vi "Initialize_Map.vi"(0 "Object_Data_In":T1, 5 "Default_Data":map{string, refnum<class "Calculator.lvclass">}(c390), 9 "Class_Names":string[](array[string])) -> (4 "Object_Data_Out":T1)   [LabVIEW 2021]
doc: "Used to initialize the map"
uses:
  Classes/Calculator/Calculator.lvclass
  Controls/Object_Data.ctl
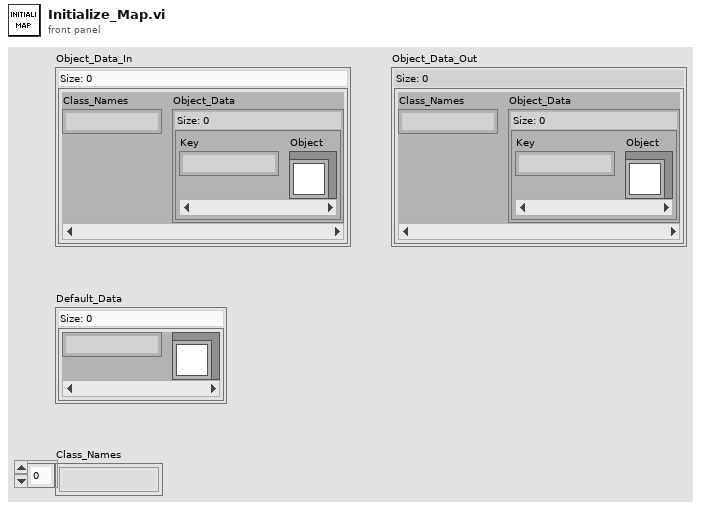
[diagram p1: front panel]
types:
  T1 = typedef "Object_Data.ctl" = map{string, map{string, refnum<class "Calculator.lvclass">}}
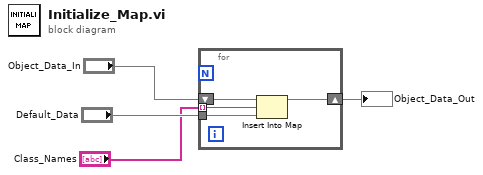
[diagram p0: block diagram]
diagram:
  n1 = for {
    tunnel: "Class_Names" -> [w8] mode=indexing
    tunnel: "Default_Data" -> [w7]
    shift-right: [w6] -> w3
    shift-left: "Object_Data_In" -> [w5]
    n2 = Insert Into Map(map in=w5, key=w8, value=w7) -> (map out=w6:T1)  [unwired: 2 out]
  }
  "Object_Data_Out" <- w3
